vi "Read baudRate.vi"(8 "error in (no error)":errorcluster, 11 "OrionBMSClass.lvclass":refnum<class "OrionBMSClass.lvclass">) -> (0 "error out":errorcluster, 2 "baudRate":T1(ring), 3 "OrionBMSClass.lvclass 2":refnum<class "OrionBMSClass.lvclass">)   [LabVIEW 2018, in "OrionBMSClass.lvclass"]
uses:
  OrionBMSClass.lvclass
  OrionBMSClass.lvclass/OrionBMSClass.ctl
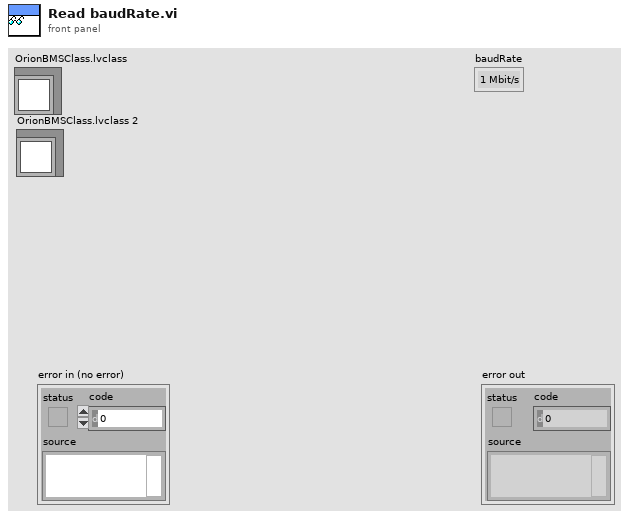
[diagram p1: front panel]
types:
  T1 = enum32{"1 Mbit/s", "800 kbit/s", "500 kbit/s", "250 kbit/s", "125 kbit/s", "50 kbit/s", "20 kbit/s", "10 kbit/s", ""}
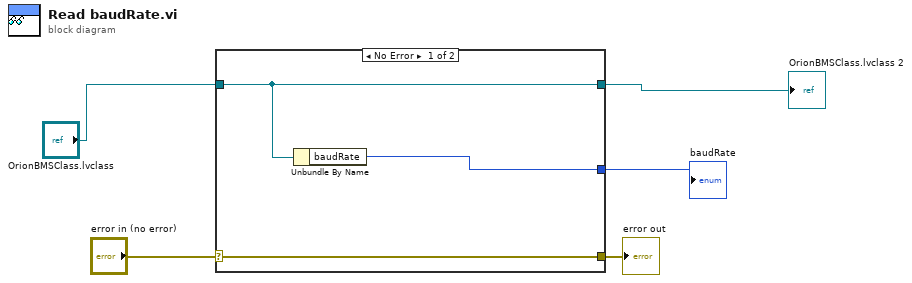
[diagram p0: block diagram]
diagram:
  n1 = case shown="No Error" "error in (no error)" {
    selector: "error in (no error)" -> [w8 w9]
    tunnel: [w8 w9] -> w4
    tunnel: [w7 w10] -> w1
    tunnel: "OrionBMSClass.lvclass" -> [w7 w10]
    tunnel: [w6 _] -> w3
    frame No Error {
      n2 = Unbundle By Name(w7) -> ("baudRate"=w6:T1)
    }
    frame Error {
    }
  }
  "error out" <- w4
  "OrionBMSClass.lvclass 2" <- w1
  "baudRate" <- w3
